vi "CheckForOxford.vi"(0 "VISA session":refnum<visa-resource-name>, 1 "search string":string, 2 "error in (no error)":errorcluster) -> (3 "dup VISA session":refnum<visa-resource-name>, 4 "String Read":string, 5 "Instrument detected":bool, 6 "error out":errorcluster)   [LabVIEW 2021]
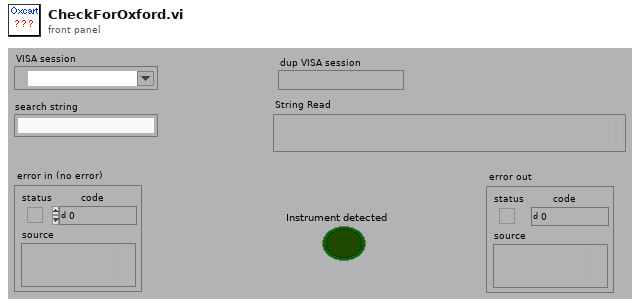
[diagram p1: front panel]
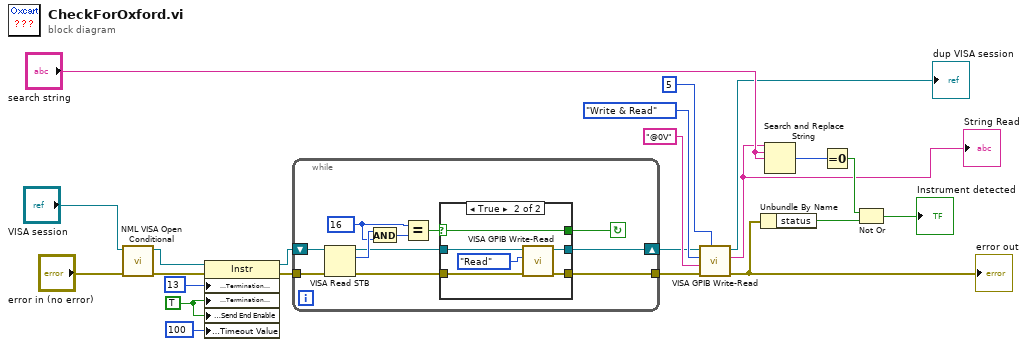
[diagram p0: block diagram]
diagram:
  w3 = TRUE ("Message Based Settings:Termination Character Enable")
  n1 = call "NML VISA Open Conditional.vi"("error in (no error)"="error in (no error)", "VISA resource name"="VISA session") -> ("error out"=w7:errorcluster, "dup VISA Session"=w8:refnum<visa-resource-name>)  [unwired: 7 in, 1 out]
  n2 = property class="Instr"(reference=w8, error in=w7, "Message Based Settings:Termination Character"=u8 13, "Message Based Settings:Termination Character Enable"=w3, "Message Based Settings:Send End Enable"=w3, "General Settings:Timeout Value"=u32 100) -> (reference out=w6:refnum<visa-resource-name>, error out=w1:errorcluster)
  n3 = while {
    tunnel: w1 -> [w30]
    tunnel: [w23] -> w4
    shift-right: [w28] -> w5
    shift-left: w6 -> [w31]
    stop <- w29 continue-if-true
    w26 = u16 16 ("y")
    n4 = VISA Read STB(8:w30, 11:w31) -> (0:w24:errorcluster, 2:w33:u16, 3:w32:refnum<visa-resource-name>)
    n5 = And(x=w33, y=w26) -> (x .and. y?=w27:u16)
    n6 = Equal?(x=w26, y=w27) -> (x = y?=w25:bool)
    n7 = case shown="True" w25 {
      selector: w25 -> [w36 w40]
      tunnel: w32 -> [w35 w41]
      tunnel: [w36 w40] -> w29
      tunnel: [w35 w39] -> w28
      tunnel: w24 -> [w34 w38]
      tunnel: [w34 w37] -> w23
      frame False {
      }
      frame True {
        n8 = call "VISA GPIB Write-Read.vi"("error in (no error)"=w38, "Action"=enum16{"Write", "Read", "Write & Read"}."Read", "VISA resource name"=w41) -> ("error out"=w37:errorcluster, "dup VISA Session"=w39:refnum<visa-resource-name>)  [unwired: 5 in, 2 out]
      }
    }
  }
  n9 = call "VISA GPIB Write-Read.vi"("Wait (ms)"=u32 5 ("wait (mS)"), "error in (no error)"=w4, "Command"="@0V" ("String to Write"), "Action"=enum16{"Write", "Read", "Write & Read"}."Write & Read", "VISA resource name"=w5) -> ("error out"=w16:errorcluster, "String Returned"=w13:string, "dup VISA Session"=→"dup VISA session":refnum<visa-resource-name>)  [unwired: 3 in, 1 out]
  "error out" <- w16
  "String Read" <- w13
  n10 = Unbundle By Name(w16) -> ("status"=w10:bool)
  n11 = Search and Replace String(input string=w13, search string="search string", replace string="search string") -> (number of replacements=w12:i32)  [unwired: 5 in, 3 out]
  n12 = Equal To 0?(x=w12) -> (x = 0?=w15:bool)
  n13 = Not Or(1:w10, 2:w15) -> (0:→"Instrument detected":bool)
